vi "Sim flow temp pressure for v2.2.vi"(10 "Offset":dbl, 11 "Spectral Amplitude":dbl) -> (3 "Array of Clusters":cluster{"[0]":dbl, "[1]":dbl, "[2]":dbl}[](array[cluster]))   [LabVIEW 2018]
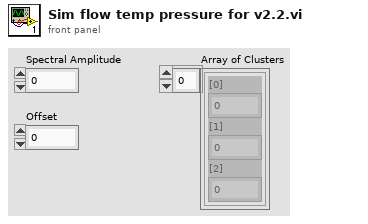
[diagram p1: front panel]
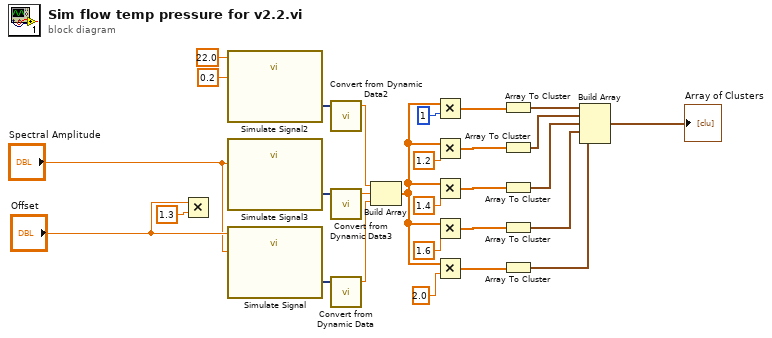
[diagram p0: block diagram]
diagram:
  n1 = Multiply(x="Offset", y=1.3) -> ()  [unwired: 1 out]
  n2 = call "Simulate Signal2"("Offset"=22.0, "Spectral amplitude"=0.2) -> ("DC Temperature Signal"=w14:dynamicdata)  [unwired: 12 in, 1 out]
  n3 = call "Simulate Signal3"("Spectral amplitude"="Spectral Amplitude") -> ("DC Pressure Signal"=w15:dynamicdata)  [unwired: 13 in, 1 out]
  n4 = call "Simulate Signal"("Offset"="Offset", "Spectral amplitude"="Spectral Amplitude") -> ("DC Flowrate Signal"=w13:dynamicdata)  [unwired: 12 in, 1 out]
  n5 = call "Convert from Dynamic Data2"("Dynamic Data Type"=w14) -> ("Scalar"=w9:dbl)  [unwired: 3 in]
  n6 = call "Convert from Dynamic Data3"("Dynamic Data Type"=w15) -> ("Scalar"=w8:dbl)  [unwired: 3 in]
  n7 = call "Convert from Dynamic Data"("Dynamic Data Type"=w13) -> ("Scalar"=w7:dbl)  [unwired: 3 in]
  n8 = Build Array(w9, w8, w7) -> (w4:dbl[])
  n9 = Multiply(x=w4, y=1) -> (x*y=w18:dbl[])
  n10 = Multiply(x=w4, y=1.2) -> (x*y=w19:dbl[])
  n11 = Multiply(x=w4, y=1.4) -> (x*y=w20:dbl[])
  n12 = Multiply(x=w4, y=1.6) -> (x*y=w21:dbl[])
  n13 = Multiply(x=w4, y=2.0) -> (x*y=w22:dbl[])
  n14 = Array To Cluster(array=w18) -> (cluster=w23:cluster{"[0]":dbl, "[1]":dbl, "[2]":dbl})
  n15 = Array To Cluster(array=w19) -> (cluster=w24:cluster{"[0]":dbl, "[1]":dbl, "[2]":dbl})
  n16 = Array To Cluster(array=w20) -> (cluster=w25:cluster{"[0]":dbl, "[1]":dbl, "[2]":dbl})
  n17 = Array To Cluster(array=w21) -> (cluster=w26:cluster{"[0]":dbl, "[1]":dbl, "[2]":dbl})
  n18 = Array To Cluster(array=w22) -> (cluster=w27:cluster{"[0]":dbl, "[1]":dbl, "[2]":dbl})
  n19 = Build Array(w23, w24, w25, w26, w27) -> (→"Array of Clusters":cluster{"[0]":dbl, "[1]":dbl, "[2]":dbl}[])
